vi "Determine Mode.vi"(8 "error in (no error)":errorcluster, 11 "DIG_IO in":refnum<class "DIG_IO.lvclass">) -> (0 "error out":errorcluster, 3 "DIG_IO out":refnum<class "DIG_IO.lvclass">)   [LabVIEW 2019, in "DIG_IO.lvlib" / "DIG_IO.lvclass"]
uses:
  Library/DIG_IO.lvclass
  Library/DIG_IO.lvclass/DIG_IO.ctl
  Custom Controls/IO Mode.ctl
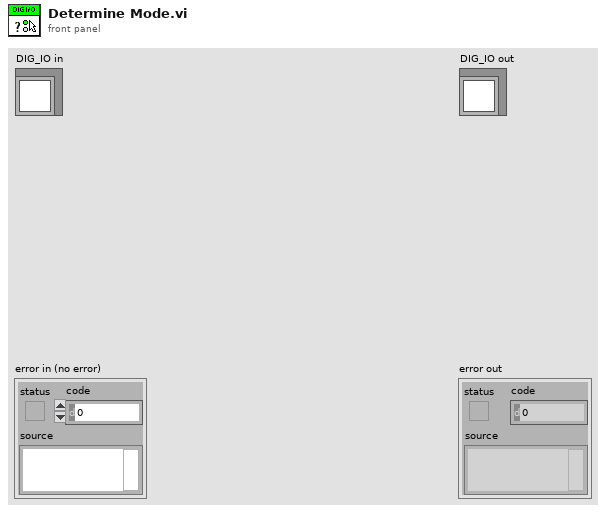
[diagram p1: front panel]
types:
  T1 = typedef "DIG_IO.lvlib/DIG_IO.lvclass/IO Mode.ctl" = enum16{"IO", "IN", "OUT"}
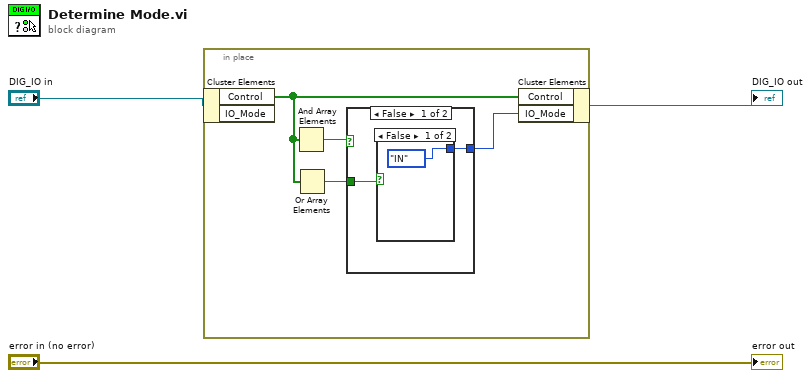
[diagram p0: block diagram]
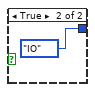
[diagram p2: hidden frame]
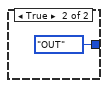
[diagram p3: hidden frame]
diagram:
  n1 = in-place {
    n2 = in-place-cluster #1("DIG_IO in") -> ("Control"=w7:bool[])  [unwired: 1 out]
    n3 = And Array Elements(Boolean array=w7) -> (logical AND=w6:bool)
    n4 = Or Array Elements(Boolean array=w7) -> (logical OR=w4:bool)
    n5 = case shown="False" w6 {
      tunnel: [w8 IO_Mode."OUT" ("IO_Mode")] -> w5
      tunnel: w4 -> [w9 _]
      frame False {
        n6 = case shown="False" w9 {
          tunnel: [IO_Mode."IN" ("IO_Mode") IO_Mode."IO" ("IO_Mode")] -> w8
          frame False {
          }
          frame True {
          }
        }
      }
      frame True {
      }
    }
    n7 = in-place-cluster #1("Control"=w7, "IO_Mode"=w5) -> (→"DIG_IO out":refnum<class "DIG_IO.lvclass">)
  }
  "error out" <- "error in (no error)"
